vi "Do Operations - Use Dynamic Dispatch Method - ArrayOfClusters.vi"(8 "error in (no error)":errorcluster, 11 "Array":T1(array[cluster])) -> (0 "error out":errorcluster, 3 "output array":T1(array[cluster]))   [LabVIEW 2011]
uses:
  ClassDefinitions/SimpleClassWithMethods/SimpleArithmetic.lvclass
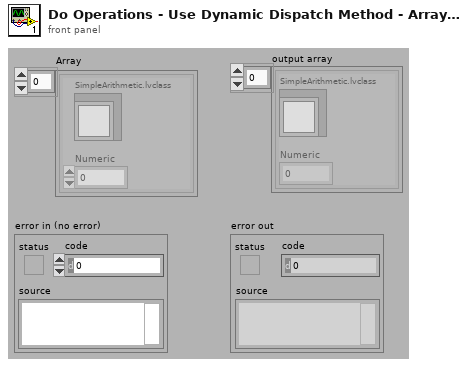
[diagram p1: front panel]
types:
  T1 = cluster{"SimpleArithmetic.lvclass":refnum<class "SimpleArithmetic.lvclass">, "Numeric":dbl}[]
  T2 = cluster{"SimpleArithmetic.lvclass":refnum<class "SimpleArithmetic.lvclass">, "Numeric":dbl}
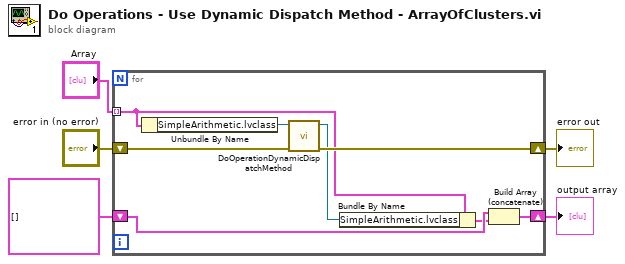
[diagram p0: block diagram]
diagram:
  n1 = for {
    tunnel: "Array" -> [w8] mode=indexing
    shift-right: [w10] -> w1
    shift-left: T1 [] ("Array") -> [w12]
    shift-right: [w11] -> w4
    shift-left: "error in (no error)" -> [w13]
    n2 = Unbundle By Name(w8) -> ("SimpleArithmetic.lvclass"=w9:refnum<class "SimpleArithmetic.lvclass">)
    n3 = call-dynamic "DoOperationDynamicDispatchMethod.vi"("error in (no error)"=w13, "SimpleArithmetic in"=w9) -> ("error out"=w11:errorcluster, "SimpleArithmetic out"=w6:refnum<class "SimpleArithmetic.lvclass">)  [unwired: 8 in]
    n4 = Bundle By Name(cluster=w8, "SimpleArithmetic.lvclass"=w6) -> (w7:T2)
    n5 = Build Array (concatenate)(w12, w7) -> (w10:T1)
  }
  "error out" <- w4
  "output array" <- w1
